vi "Change ILC Mode.vi"(8 "error in (no error)":errorcluster, 9 "Command.ILCMode":u16, 10 "DesktopModbus in":refnum<class "DesktopModbus.lvclass">, 11 "FAILC in":refnum<class "FAILC.lvclass">) -> (0 "error out":errorcluster, 2 "DesktopModbus out":refnum<class "DesktopModbus.lvclass">, 3 "FAILC out":refnum<class "FAILC.lvclass">)   [LabVIEW 2016]
uses:
  Model/Modbus/DesktopModbus/DesktopModbus.lvclass
  Common_RT_FAILC/FAILC/FAILC.lvclass
  D:/Code/ts_FAMT/Common_RT_ILC/ILC/ILC.lvclass
  Common_RT_ILC/ILC/ILC.lvclass/ILC.ctl
  Common_RT_Modbus/DynamicFrameParser/DynamicFrameParser.lvclass
  Common_RT_ILC/ILC/ILC.lvclass
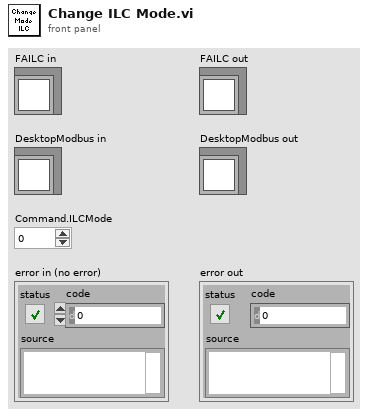
[diagram p1: front panel]
types:
  T1 = typedef "RTILC.lvlib/ILCData.ctl" = cluster{"Constants":T2, "Command":T3, "Telemetry":T5, "Responses":T6}
  T2 = typedef "RTILC.lvlib/ILCConstants.ctl" = cluster{"Subnet":u8, "Address":u8}
  T3 = typedef "RTILC.lvlib/ILCCommand.ctl" = cluster{"ILCMode":u16, "TemporaryAddress":u8, "ADCScanRate":T4, "ADCChannel":u8, "ADCOffset":sgl, "ADCSensitivity":sgl}
  T4 = typedef "RTILC.lvlib/ILCScanRates.ctl" = u8
  T5 = typedef "RTILC.lvlib/ILCTelemetry.ctl" = cluster{"UniqueID":u64, "FirmwareType":u8, "NetworkNodeType":u8, "ILCOption":u8, "NetworkNodeOption":u8, "MajorRevision":u8, "MinorRevision":u8, "FirmwareName":string, "ILCMode":u16, "MajorFault":bool, "MinorFault":bool, "FaultOverride":bool, "UniqueIDCRCMismatch":bool, "AppTypeNodeTypeMismatch":bool, "AppMissing":bool, "AppCRCMismatch":bool, "TEDSNotFound":bool, "TEDS1Mismatch":bool, "TEDS2Mismatch":bool, "WatchdogResetDetected":bool, "BrownoutDetected":bool, "EventTrapResetDetected":bool, "TemporaryAddress":u8, "ADCScanRate":T4, "DAC1":u16, "DAC2":u16, "DAC3":u16, "DAC4":u16, "MainADCCalibrationK":sgl[], "MainSensorOffset":sgl[], "MainSensorSensitivity":sgl[], "BackupADCCalibrationK":sgl[], "BackupSensorOffset":sgl[], "BackupSensorSensitivity":sgl[]}
  T6 = typedef "RTILC.lvlib/ILCResponses.ctl" = cluster{"ReportServerID":T7, "ReportServerStatus":T7, "ILCMode":T7, "SetTemporaryAddress":T7, "Reset":T7, "ADCScanRate":T7, "ADCOffsetSensitivity":T7, "ReadDAC":T7, "ReadCalibration":T7}
  T7 = typedef "RTModbus.lvlib/ExceptionCodes.ctl" = u16
  T8 = typedef "RTModbus.lvlib/Frame.ctl" = cluster{"Data":u8[], "WaitForTrigger":bool, "WaitForRx":u16, "TriggerIRQ":bool, "DelayTicks":u16, "DelayMicroseconds":u16, "DelayMilliseconds":u16}
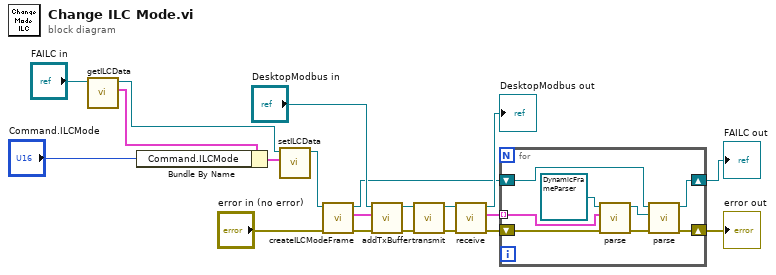
[diagram p0: block diagram]
diagram:
  n1 = call "getILCData.vi"("ILC in"="FAILC in") -> ("ILCData"=w1:T1, "ILC out"=w4:refnum<class "FAILC.lvclass">)  [unwired: 9 in]
  n2 = Bundle By Name(cluster=w1, "Command.ILCMode"="Command.ILCMode") -> (w2:T1)
  n3 = call "setILCData.vi"("ILCData"=w2, "ILC in"=w4) -> ("ILC out"=w5:refnum<class "FAILC.lvclass">)  [unwired: 9 in]
  n4 = call "createILCModeFrame.vi"("error in (no error)"="error in (no error)", "ILC in"=w5) -> ("error out"=w8:errorcluster, "Frame"=w6:T8, "ILC out"=w13:refnum<class "FAILC.lvclass">)  [unwired: 7 in]
  n5 = call-dynamic "addTxBuffer.vi"("error in (no error)"=w8, "Frame"=w6, "DesktopModbus in"="DesktopModbus in") -> ("error out"=w9:errorcluster, "DesktopModbus out"=w7:refnum<class "DesktopModbus.lvclass">)  [unwired: 7 in]
  n6 = call-dynamic "transmit.vi"("error in (no error)"=w9, "DesktopModbus in"=w7) -> ("error out"=w10:errorcluster, "DesktopModbus out"=w11:refnum<class "DesktopModbus.lvclass">)  [unwired: 8 in]
  n7 = call-dynamic "receive.vi"("error in (no error)"=w10, "DesktopModbus in"=w11) -> ("error out"=w14:errorcluster, "Data"=w12:T8[], "DesktopModbus out"=→"DesktopModbus out":refnum<class "DesktopModbus.lvclass">)  [unwired: 7 in]
  n8 = for {
    tunnel: w12 -> [w28] mode=indexing
    shift-right: [w24] -> w16
    shift-left: w13 -> [w25]
    shift-right: [w21] -> w20
    shift-left: w14 -> [w22]
    n9 = call "parse.vi"("error in (no error)"=w22, "Frame"=w28, "FrameParser in"=refnum<class "DynamicFrameParser.lvclass"> refnum ("RTModbus.lvlib:DynamicFrameParser.lvclass")) -> ("error out"=w23:errorcluster, "FrameParser out"=w26:refnum<class "DynamicFrameParser.lvclass">)  [unwired: 7 in]
    n10 = call-dynamic "parse.vi"("error in (no error)"=w23, "DynamicFrameParser"=w26, "FAILC in"=w25) -> ("error out"=w21:errorcluster, "FAILC out"=w24:refnum<class "FAILC.lvclass">)  [unwired: 6 in, 1 out]
  }
  "error out" <- w20
  "FAILC out" <- w16
